vi "Arrange Panel.vi"(8 "error in (no error)":errorcluster, 10 "Shift?":bool, 11 "VI Refnum in":refnum<vi>) -> (0 "error out":errorcluster, 3 "VI Refnum out":refnum<vi>)   [LabVIEW 2019, in "Builtins.lvlib"]
doc: "Arranges the selected controls to the panel grid by left or top edges (hold shift). If nothing is selected, this will arrange all the controls on the panel into columns with a dead zone offset from the panel origin.\n\nCreated by: Ryan Pacini"
uses:
  Builtins.lvlib
  Align.ctl
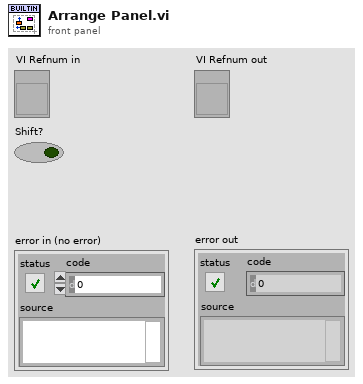
[diagram p1: front panel]
types:
  T1 = typedef "Builtins.lvlib/Align.ctl" = enum8{"Top Edges", "Vertical Centers", "Bottom Edges", "Left Edges", "Horizontal Centers", "Right Edges"}
  T2 = typedef "LVRectTypeDef.ctl" = cluster{"Left":i16, "Top":i16, "Right":i16, "Bottom":i16}
  T3 = cluster{"Left":i16, "Top":i16, "Right":i16, "Bottom":i16}[]
  T4 = enum32{"invalid VI type", "Standard VI", "Control VI", "Global VI", "Polymorphic VI", "Configuration VI", "SubSystem", "Facade VI", "Method VI", "Statechart Diagram VI"}
  T5 = cluster{"Left":i16, "Top":i16, "Right":i16, "Bottom":i16}[][]
  T6 = cluster{"Top":i16, "MasterRect":T2, refnum<vi>}[]
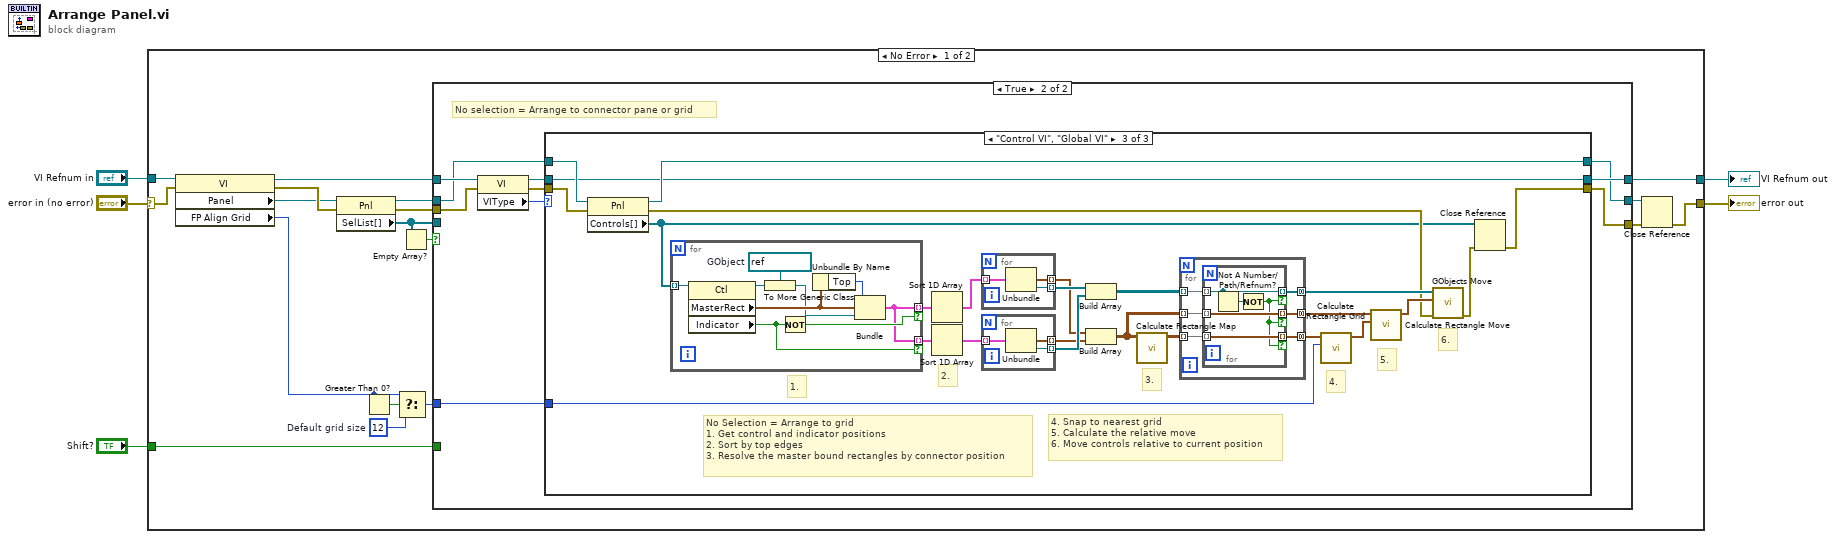
[diagram p0: block diagram]
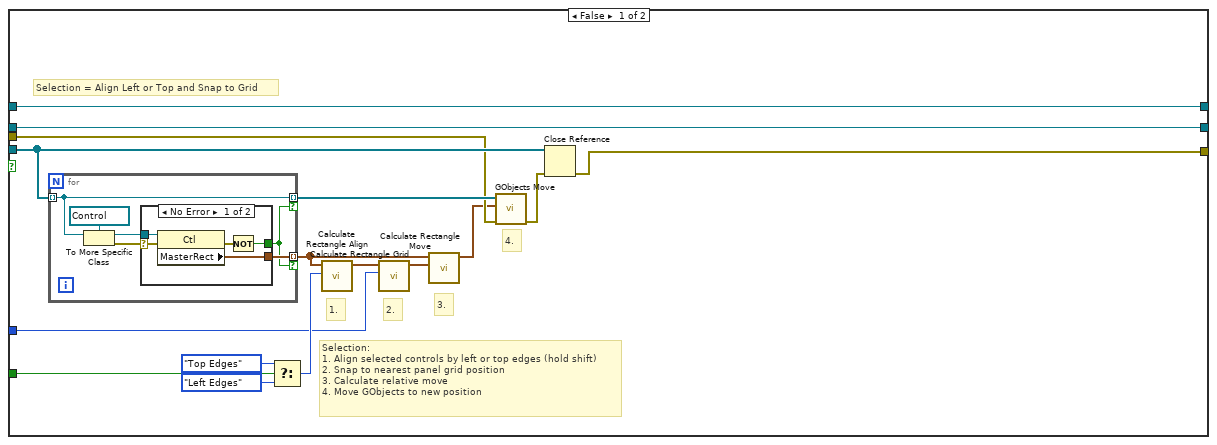
[diagram p2: hidden frame]
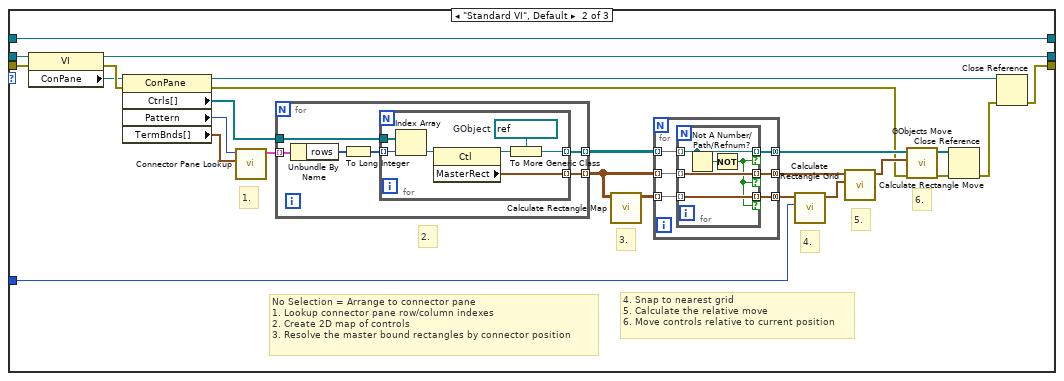
[diagram p5: hidden frame]
diagram:
  n1 = case shown="No Error" "error in (no error)" {
    selector: "error in (no error)" -> [w22 w164]
    tunnel: "VI Refnum in" -> [w23 w165]
    tunnel: [w9 w165] -> w4
    tunnel: [w18 w164] -> w2
    tunnel: "Shift?" -> [w6 _]
    frame No Error {
      w13 = 12  # Default grid size
      n2 = property class="VI"(reference=w23, error in=w22) -> (reference out=w10:refnum<vi>, error out=w21:errorcluster, "Panel"=w20:refnum<vi>, "FP Align Grid"=w12:i32)
      n3 = property class="Pnl"(reference=w20, error in=w21) -> (reference out=w8:refnum<vi>, error out=w16:errorcluster, "SelList[]"=w17:refnum<vi>[])
      n4 = Greater Than 0?(x=w12) -> (x > 0?=w14:bool)
      n5 = Select(t=w12, s=w14, f=w13) -> (s? t:f=w11:i32)
      n6 = Empty Array?(array=w17) -> (empty?=w15:bool)
      n7 = case shown="True" w15 {
        tunnel: [w39 w57] -> w19
        tunnel: w17 -> [w36 _]
        tunnel: w16 -> [w32 w55]
        tunnel: w11 -> [w29 w58]
        tunnel: w6 -> [w30 _]
        tunnel: w10 -> [w25 w60]
        tunnel: [w25 w59] -> w9
        tunnel: w8 -> [w24 w52]
        tunnel: [w24 w51] -> w7
        frame False {
          # "3."
          # "Selection:\n1. Align selected controls by left or top edges (hold shift)\n2. Snap to nearest panel grid position\n3. Calculate relative move\n4. Move GObjects to new position"
          # "2."
          # "4."
          # "1."
          # "Selection = Align Left or Top and Snap to Grid"
          n8 = for {
            tunnel: w36 -> [w40] mode=indexing
            tunnel: [w40] -> w38 mode=indexing if=w41
            tunnel: [w44] -> w28 mode=indexing if=w41
            n9 = To More Specific Class(target class=refnum<vi> refnum, reference=w40) -> (specific class reference=w42:refnum<vi>, error out=w43:errorcluster)  [unwired: 1 in]
            n10 = case shown="No Error" w43 {
              selector: w43 -> [w49 _]
              tunnel: [w50 _] -> w44
              tunnel: w42 -> [w48 _]
              tunnel: [w47 _] -> w41
              frame No Error {
                n11 = property class="Ctl"(reference=w48, error in=w49) -> (error out=w46:errorcluster, "MasterRect"=w50:T2)  [unwired: 1 out]
                n12 = Not(x=w46) -> (.not. x?=w47:bool)
              }
              frame Error {
              }
            }
          }
          n13 = Select(t=Align."Top Edges" ("Align Type"), s=w30, f=Align."Left Edges" ("Align Type")) -> (s? t:f=w33:T1)
          n14 = call "Calculate Rectangle Align.vi"("Align Type"=w33, "Rects in"=w28) -> ("Resolved Rects out"=w31:T3)  [unwired: 9 in]
          n15 = call "Calculate Rectangle Grid.vi"("Grid Size (12px)"=w29, "Rects in"=w31) -> ("Resolved Rects out"=w27:T3)  [unwired: 9 in]
          n16 = call "Calculate Rectangle Move.vi"("End Rects out"=w27, "Start Rects in"=w28) -> ("Relative Move"=w26:cluster{"Left":i32, "Top":i32}[])  [unwired: 9 in]
          n17 = call "GObjects Move.vi"("error in (no error)"=w32, "Relative Moves in"=w26, "GObjects in"=w38) -> ("error out"=w37:errorcluster)  [unwired: 7 in, 1 out]
          n18 = Close Reference(reference=w36, error in (no error)=w37) -> (error out=w39:errorcluster)
        }
        frame True {
          # "No selection = Arrange to connector pane or grid"
          n19 = property class="VI"(reference=w60, error in=w55) -> (reference out=w56:refnum<vi>, error out=w54:errorcluster, "VIType"=w53:T4)
          n20 = case shown="\"Control VI\", \"Global VI\"" w53 {
            tunnel: [w62 w86 w125] -> w59
            tunnel: w58 -> [_ w78 w134]
            tunnel: [w63 w67 w123] -> w57
            tunnel: w56 -> [w62 w66 w125]
            tunnel: w54 -> [w63 w65 w128]
            tunnel: w52 -> [w61 w64 w126]
            tunnel: [w61 w64 w127] -> w51
            frame "invalid VI type", "Polymorphic VI" {
            }
            frame "Standard VI", Default {
              # "No Selection = Arrange to connector pane\n1. Lookup connector pane row/column indexes\n2. Create 2D map of controls\n3. Resolve the master bound rectangles by connector position"
              # "3."
              # "2."
              # "1."
              # "5."
              # "4."
              # "4. Snap to nearest grid\n5. Calculate the relative move\n6. Move controls relative to current position"
              # "6."
              n21 = property class="VI"(reference=w66, error in=w65) -> (reference out=w86:refnum<vi>, error out=w85:errorcluster, "ConPane"=w84:refnum<vi>)
              n22 = property class="ConPane"(reference=w84, error in=w85) -> (reference out=w70:refnum<vi>, error out=w69:errorcluster, "Ctrls[]"=w83:refnum<vi>[], "Pattern"=w80:u32, "TermBnds[]"=w81:T2[])
              n23 = call "Connector Pane Lookup.vi"("TermBnds"=w81, "Pattern"=w80) -> ("columns"=w82:cluster{"rows":u8[]}[])  [unwired: 9 in]
              n24 = for {
                tunnel: [w105] -> w75 mode=indexing
                tunnel: w83 -> [w104]
                tunnel: w82 -> [w103] mode=indexing
                tunnel: [w100] -> w77 mode=indexing
                n25 = Unbundle By Name(w103) -> ("rows"=w102:u8[])
                n26 = To Long Integer(number=w102) -> (32bit integer=w101:i32[])
                n27 = for {
                  tunnel: w104 -> [w111]
                  tunnel: [w112] -> w105 mode=indexing
                  tunnel: w101 -> [w109] mode=indexing
                  tunnel: [w106] -> w100 mode=indexing
                  w108 = refnum<vi> refnum  # GObject
                  n28 = Index Array(array=w111, index=w109) -> (element=w110:refnum<vi>)
                  n29 = property class="Ctl"(reference=w110) -> (reference out=w107:refnum<vi>, "MasterRect"=w112:T2)  [unwired: 1 in, 1 out]
                  n30 = To More Generic Class(target class=w108, reference=w107) -> (generic class reference=w106:refnum<vi>)
                }
              }
              n31 = call "Calculate Rectangle Map.vi"("MasterBndRects in"=w75) -> ("Resolved MasterBndRects out"=w76:T5)  [unwired: 8 in, 2 out]
              n32 = for {
                tunnel: w77 -> [w94] mode=indexing
                tunnel: w76 -> [w93] mode=indexing
                tunnel: w75 -> [w92] mode=indexing
                tunnel: [w91] -> w73 mode=concatenating
                tunnel: [w90] -> w74 mode=concatenating
                tunnel: [w89] -> w71 mode=concatenating
                n33 = for {
                  tunnel: w94 -> [w97] mode=indexing
                  tunnel: w93 -> [w98] mode=indexing
                  tunnel: w92 -> [w99] mode=indexing
                  tunnel: [w97] -> w91 mode=indexing if=w95
                  tunnel: [w99] -> w90 mode=indexing if=w95
                  tunnel: [w98] -> w89 mode=indexing if=w95
                  n34 = Not A Number/Path/Refnum?(number/path/refnum=w97) -> (NaN/Path/Refnum?=w96:bool)
                  n35 = Not(x=w96) -> (.not. x?=w95:bool)
                }
              }
              n36 = call "Calculate Rectangle Grid.vi"("Grid Size (12px)"=w78, "Rects in"=w71) -> ("Resolved Rects out"=w79:T3)  [unwired: 9 in]
              n37 = call "Calculate Rectangle Move.vi"("End Rects out"=w79, "Start Rects in"=w74) -> ("Relative Move"=w87:cluster{"Left":i32, "Top":i32}[])  [unwired: 9 in]
              n38 = call "GObjects Move.vi"("error in (no error)"=w69, "Relative Moves in"=w87, "GObjects in"=w73) -> ("error out"=w88:errorcluster, "GObjects out"=w72:refnum<vi>[])  [unwired: 7 in]
              n39 = Close Reference(reference=w72, error in (no error)=w88) -> (error out=w68:errorcluster)
              n40 = Close Reference(reference=w70, error in (no error)=w68) -> (error out=w67:errorcluster)
            }
            frame "Control VI", "Global VI" {
              # "1."
              # "2."
              # "No Selection = Arrange to grid\n1. Get control and indicator positions\n2. Sort by top edges\n3. Resolve the master bound rectangles by connector position"
              # "3."
              # "5."
              # "4."
              # "4. Snap to nearest grid\n5. Calculate the relative move\n6. Move controls relative to current position"
              # "6."
              n41 = property class="Pnl"(reference=w126, error in=w128) -> (reference out=w127:refnum<vi>, error out=w129:errorcluster, "Controls[]"=w124:refnum<vi>[])
              n42 = for {
                tunnel: w124 -> [w152] mode=indexing
                tunnel: [w145] -> w122 mode=indexing if=w146
                tunnel: [w145] -> w121 mode=indexing if=w144
                w148 = refnum<vi> refnum  # GObject
                n43 = property class="Ctl"(reference=w152) -> (reference out=w149:refnum<vi>, "MasterRect"=w151:T2, "Indicator"=w144:bool)  [unwired: 1 in, 1 out]
                n44 = To More Generic Class(target class=w148, reference=w149) -> (generic class reference=w147:refnum<vi>)
                n45 = Not(x=w144) -> (.not. x?=w146:bool)
                n46 = Unbundle By Name(w151) -> ("Top"=w150:i16)
                n47 = Bundle("Top"=w150, "MasterRect"=w151, w147) -> (w145:cluster{"Top":i16, "MasterRect":T2, refnum<vi>})  [unwired: 1 in]
              }
              n48 = Sort 1D Array(array=w122) -> (sorted array=w120:T6)
              n49 = Sort 1D Array(array=w121) -> (sorted array=w119:T6)
              n50 = for {
                tunnel: w120 -> [w143] mode=indexing
                tunnel: [w142] -> w116 mode=indexing
                tunnel: [w141] -> w118 mode=indexing
                n51 = Unbundle(w143) -> ("MasterRect"=w142:T2, w141:refnum<vi>)  [unwired: 1 out]
              }
              n52 = for {
                tunnel: w119 -> [w140] mode=indexing
                tunnel: [w139] -> w115 mode=indexing
                tunnel: [w138] -> w117 mode=indexing
                n53 = Unbundle(w140) -> ("MasterRect"=w139:T2, w138:refnum<vi>)  [unwired: 1 out]
              }
              n54 = Build Array(w118, w117) -> (w113:refnum<vi>[][])
              n55 = Build Array(w116, w115) -> (w114:T2[][])
              n56 = call "Calculate Rectangle Map.vi"("MasterBndRects in"=w114) -> ("Resolved MasterBndRects out"=w133:T5)  [unwired: 8 in, 2 out]
              n57 = for {
                tunnel: w113 -> [w158] mode=indexing
                tunnel: w133 -> [w157] mode=indexing
                tunnel: w114 -> [w156] mode=indexing
                tunnel: [w155] -> w131 mode=concatenating
                tunnel: [w154] -> w132 mode=concatenating
                tunnel: [w153] -> w130 mode=concatenating
                n58 = for {
                  tunnel: w158 -> [w161] mode=indexing
                  tunnel: w157 -> [w162] mode=indexing
                  tunnel: w156 -> [w163] mode=indexing
                  tunnel: [w161] -> w155 mode=indexing if=w159
                  tunnel: [w163] -> w154 mode=indexing if=w159
                  tunnel: [w162] -> w153 mode=indexing if=w159
                  n59 = Not A Number/Path/Refnum?(number/path/refnum=w161) -> (NaN/Path/Refnum?=w160:bool)
                  n60 = Not(x=w160) -> (.not. x?=w159:bool)
                }
              }
              n61 = call "Calculate Rectangle Grid.vi"("Grid Size (12px)"=w134, "Rects in"=w130) -> ("Resolved Rects out"=w135:T3)  [unwired: 9 in]
              n62 = call "Calculate Rectangle Move.vi"("End Rects out"=w135, "Start Rects in"=w132) -> ("Relative Move"=w136:cluster{"Left":i32, "Top":i32}[])  [unwired: 9 in]
              n63 = call "GObjects Move.vi"("error in (no error)"=w129, "Relative Moves in"=w136, "GObjects in"=w131) -> ("error out"=w137:errorcluster)  [unwired: 7 in, 1 out]
              n64 = Close Reference(reference=w124, error in (no error)=w137) -> (error out=w123:errorcluster)
            }
          }
        }
      }
      n65 = Close Reference(reference=w7, error in (no error)=w19) -> (error out=w18:errorcluster)
    }
    frame Error {
    }
  }
  "VI Refnum out" <- w4
  "error out" <- w2
